vi "check_simulator_version.vi"(8 "error in":errorcluster, 11 "Response JSON":string) -> (0 "error out":errorcluster, 2 "Simulator Version":i32[](array[numeric]), 3 "Compatible":bool)   [LabVIEW 2019]
doc: "Check compatibility between the simulator's version and the client's version."
panel:
  in  "Client Version":string="1.13.1"
  in  "Client API Version":string="5.0"
  out "API Version":i32[](array[numeric])
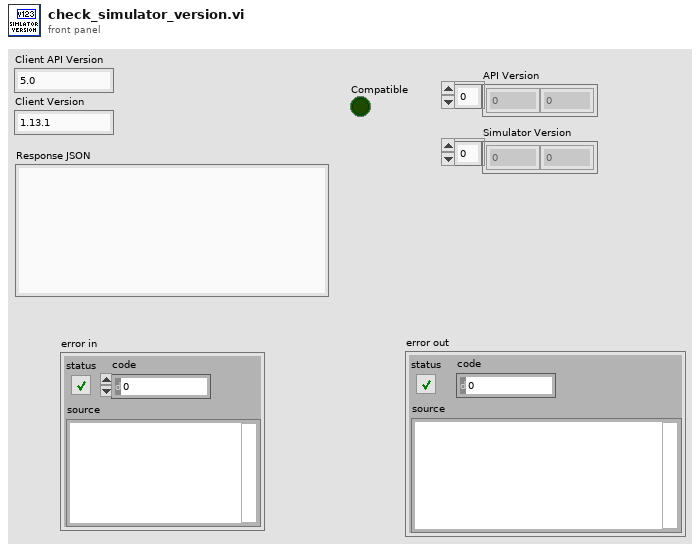
[diagram p1: front panel]
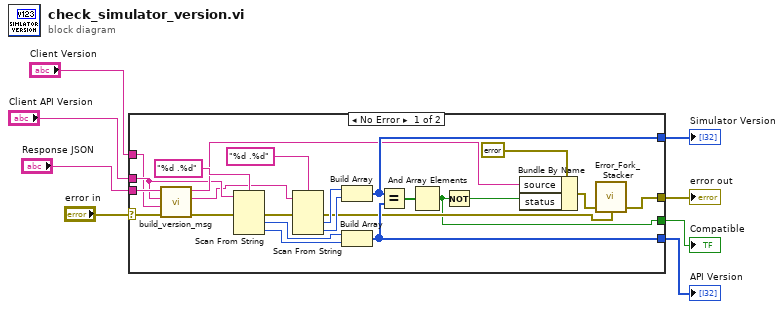
[diagram p0: block diagram]
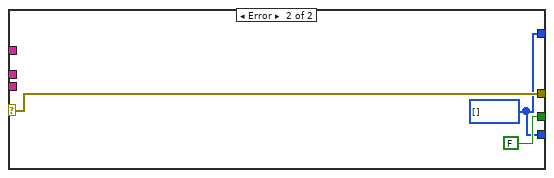
[diagram p2: hidden frame]
diagram:
  n1 = case shown="No Error" "error in" {
    selector: "error in" -> [w16 w34]
    tunnel: [w14 w34] -> w7
    tunnel: [w24 w32] -> w6
    tunnel: [w9 FALSE] -> w5
    tunnel: "Response JSON" -> [w18 _]
    tunnel: [w23 w32] -> w4
    tunnel: "Client Version" -> [w15 _]
    tunnel: "Client API Version" -> [w17 _]
    frame No Error {
      n2 = call "build_version_msg.vi"("error in"=w16, "Client version"=w15, "Client API version"=w17, "Response JSON"=w18) -> ("error out"=w20:errorcluster, "API version"=w11:string, "Message"=w21:string)  [unwired: 1 in]
      n3 = Scan From String(format string="%d .%d", input string=w17, error in=w20) -> (error out=w19:errorcluster, output 1=w25:i32, output 2=w22:i32)  [unwired: 3 in, 2 out]
      n4 = Scan From String(format string="%d .%d", input string=w11, error in=w19) -> (error out=w12:errorcluster, output 1=w27:i32, output 2=w26:i32)  [unwired: 3 in, 2 out]
      n5 = Build Array(w27, w26) -> (w24:i32[])
      n6 = Build Array(w25, w22) -> (w23:i32[])
      n7 = Equal?(x=w24, y=w23) -> (x = y?=w31:bool[])
      n8 = And Array Elements(Boolean array=w31) -> (logical AND=w9:bool)
      n9 = Not(x=w9) -> (.not. x?=w10:bool)
      n10 = Bundle By Name(cluster=errorcluster {"status"=TRUE, "code"=0, "source"=""} ("f"), "source"=w21, "status"=w10) -> (w13:errorcluster)
      n11 = call "Error_Fork_Stacker.vi"("Error Fork B"=w12, "Error Fork A"=w13) -> ("Error Out"=w14:errorcluster)  [unwired: 2 in]
    }
    frame Error {
      w32 = i32[] []
    }
  }
  "error out" <- w7
  "Simulator Version" <- w6
  "Compatible" <- w5
  "API Version" <- w4
